vi "display.vi"(8 "error in (no error)":errorcluster, 11 "RedheadDuck in":refnum<class "RedheadDuck.lvclass">) -> (0 "error out":errorcluster, 2 "State":string, 3 "RedheadDuck out":refnum<class "RedheadDuck.lvclass">)   [LabVIEW 2013, in "RedheadDuck.lvclass"]
uses:
  RedheadDuck.lvclass
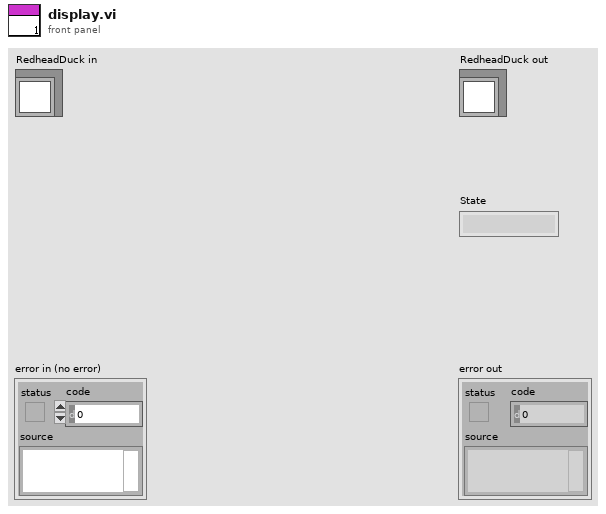
[diagram p1: front panel]
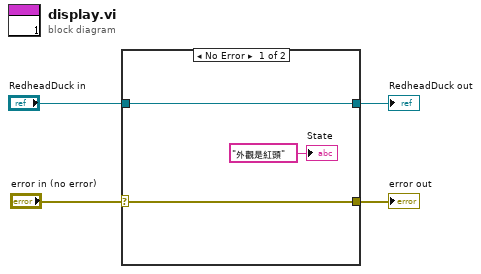
[diagram p0: block diagram]
diagram:
  n1 = case shown="No Error" "error in (no error)" {
    selector: "error in (no error)" -> [w6 w8]
    tunnel: [w7 w9] -> w3
    tunnel: "RedheadDuck in" -> [w7 w9]
    tunnel: [w6 w8] -> w1
    frame No Error {
      "State" <- "外觀是紅頭" ("State")
    }
    frame Error {
    }
  }
  "error out" <- w1
  "RedheadDuck out" <- w3
